vi "AO_Range_Min.vi"(8 "error in":errorcluster, 10 "Action":enum16{"Write", "Read"}(ring), 11 "AO | Min":dbl[](array[numeric])) -> (0 "error out":errorcluster, 3 "AO | Min":dbl[](array[numeric]))   [LabVIEW 2021]
doc: "Functional Global Variable:\n- Write the value into the memory \nor\n- Read the value from the memory"
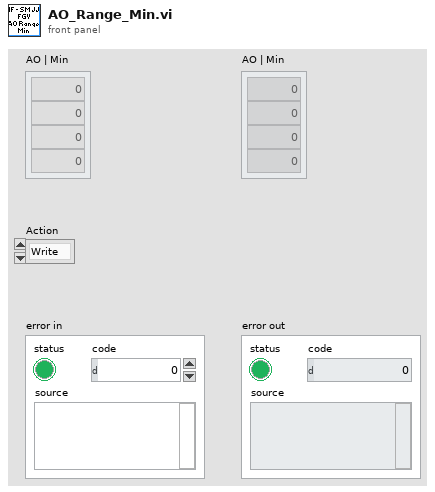
[diagram p1: front panel]
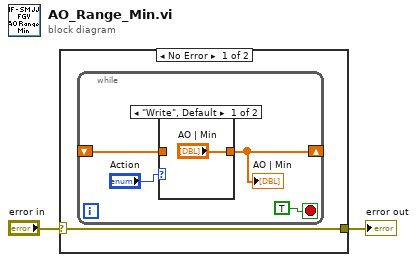
[diagram p0: block diagram]
diagram:
  n1 = case shown="No Error" "error in" {
    selector: "error in" -> [w3 w10]
    tunnel: [w3 w10] -> w1
    frame No Error {
      n2 = while {
        shift-right: [w4] -> _
        shift-left: _ -> [w5]
        stop <- TRUE stop-if-true
        n3 = case shown="\"Write\", Default" "Action" {
          tunnel: w5 -> [_ w9]
          tunnel: ["AO | Min" w9] -> w4
          frame "Write", Default {
          }
          frame "Read" {
          }
        }
        "AO | Min" <- w4
      }
    }
    frame Error {
    }
  }
  "error out" <- w1
